vi "weight.vi"(7 "python in":refnum<k35>, 8 "error in":errorcluster, 11 "List Concentration In":T1(array[cluster]) {"N. Peak" items=["0.000000", "1.000000", "2.000000", "3.000000", "4.000000", "5.000000", "6.000000", "7.000000", "8.000000", "9.000000", "10.000000", "11.000000", "12.000000", "13.000000", "14.000000", "15.000000", "16.000000", "17.000000", "18.000000", "19.000000", "20.000000", "21.000000", "22.000000", "23.000000", "24.000000", "25.000000", "26.000000", "27.000000", "28.000000"]}) -> (0 "error out":errorcluster, 3 "List Concentration Out":T1(array[cluster]) {"N. Peak" items=["0.000000", "1.000000", "2.000000", "3.000000", "4.000000", "5.000000", "6.000000", "7.000000", "8.000000", "9.000000", "10.000000", "11.000000", "12.000000", "13.000000", "14.000000", "15.000000", "16.000000", "17.000000", "18.000000", "19.000000", "20.000000", "21.000000", "22.000000", "23.000000", "24.000000", "25.000000", "26.000000", "27.000000", "28.000000"]}, 5 "python out":refnum<k35>)   [LabVIEW 2023]
uses:
  0a205a4e-a878-4401-81a0-2c59aac56441.vi
  <vilib>/Comparison/Equal/Equal Functor/Equal Functor.lvclass
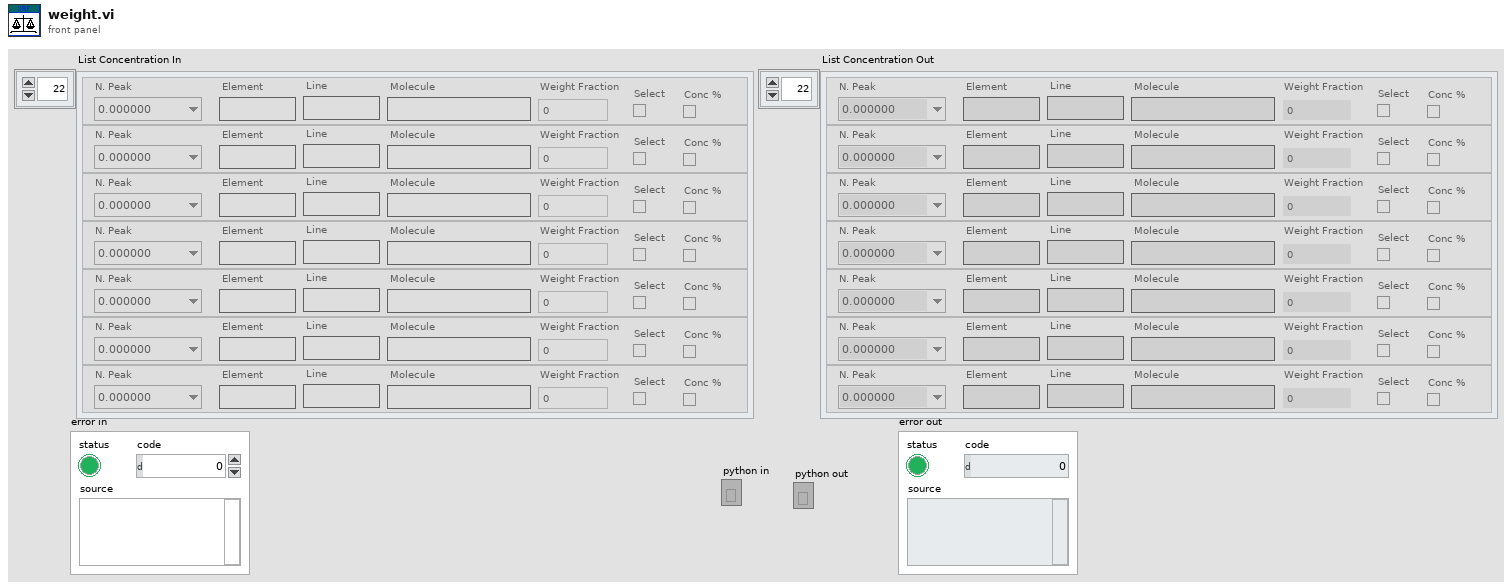
[diagram p1: front panel]
types:
  T1 = cluster{"N. Peak":u16, "Element":string, "Molecule":string, "Weight Fraction":dbl, "Select":bool, "Conc %":bool, "Line":string}[]
  T2 = cluster{"N. Peak":u16, "Element":string, "Molecule":string, "Weight Fraction":dbl, "Select":bool, "Conc %":bool, "Line":string}
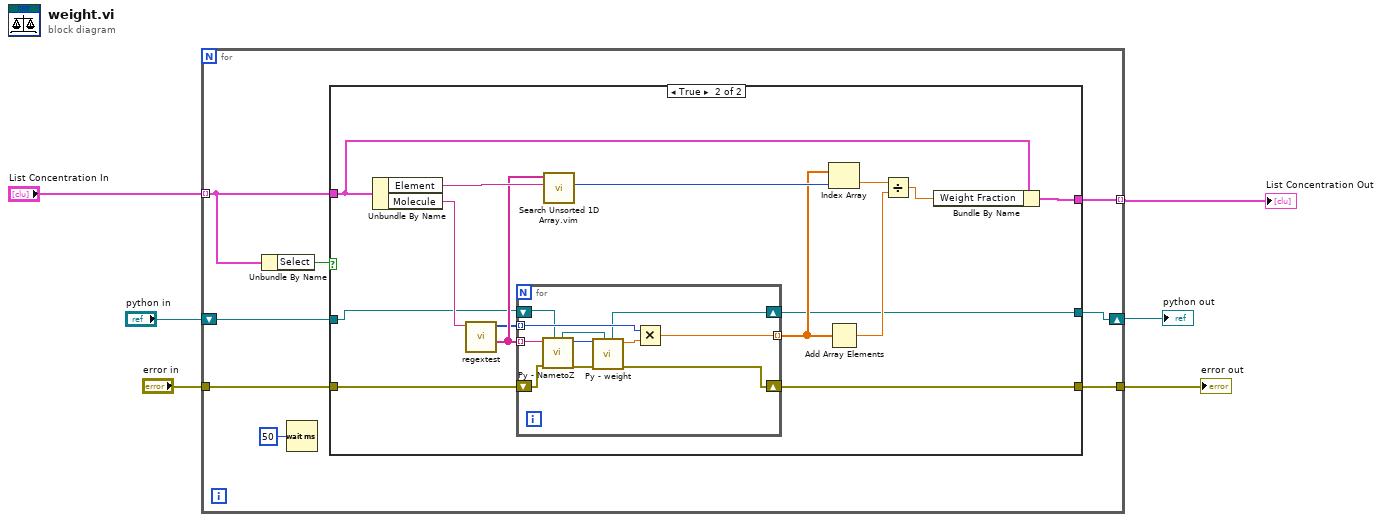
[diagram p0: block diagram]
diagram:
  n1 = for {
    tunnel: "error in" -> [w12]
    tunnel: [w13] -> w5
    tunnel: "List Concentration In" -> [w11] mode=indexing
    tunnel: [w10] -> w3 mode=indexing
    shift-right: [w8] -> w1
    shift-left: "python in" -> [w9]
    n2 = Unbundle By Name(w11) -> ("Select"=w14:bool)
    n3 = Wait (ms)(milliseconds to wait=u32 50) -> ()  [unwired: 1 out]
    n4 = case shown="True" w14 {
      tunnel: [w17 w20] -> w13
      tunnel: w12 -> [w17 w21]
      tunnel: w11 -> [w16 w32]
      tunnel: [w16 w31] -> w10
      tunnel: w9 -> [w15 w19]
      tunnel: [w15 w18] -> w8
      frame False {
      }
      frame True {
        n5 = Unbundle By Name(w32) -> ("Element"=w29:string, "Molecule"=w30:string)
        n6 = call "regextest.vi"("Molecule"=w30) -> ("Elements"=w28:string[], "Numbers"=w27:i32[])  [unwired: 8 in, 1 out]
        n7 = for {
          tunnel: w28 -> [w41] mode=indexing
          tunnel: w27 -> [w43] mode=indexing
          tunnel: [w42] -> w25 mode=indexing
          shift-right: [w37] -> w20
          shift-left: w21 -> [w38]
          shift-right: [w33] -> w18
          shift-left: w19 -> [w35]
          n8 = call "Py - NametoZ.vi"("python in"=w35, "error in"=w38, "Name Element"=w41) -> ("error out"=w36:errorcluster, "Z"=w40:i32, "python out"=w34:refnum<k35>)  [unwired: 6 in]
          n9 = call "Py - weight.vi"("python in"=w34, "error in"=w36, "Z"=w40) -> ("error out"=w37:errorcluster, "weight (g/mol)"=w39:dbl, "python out"=w33:refnum<k35>)  [unwired: 6 in]
          n10 = Multiply(x=w43, y=w39) -> (x*y=w42:dbl)
        }
        n11 = call "Search Unsorted 1D Array.vim"("element"=w29, "unsorted 1D array"=w28) -> ("index of element"=w26:i32)  [unwired: 9 in]
        n12 = Index Array(array=w25, index=w26) -> (element=w24:dbl)
        n13 = Add Array Elements(numeric array=w25) -> (sum=w23:dbl)
        n14 = Divide(x=w24, y=w23) -> (x/y=w22:dbl)
        n15 = Bundle By Name(cluster=w32, "Weight Fraction"=w22) -> (w31:T2)
      }
    }
  }
  "error out" <- w5
  "List Concentration Out" <- w3
  "python out" <- w1
